vi "Coincidence Stats Rolling Add.vi"(8 "error in (no error)":errorcluster, 10 "New data":T3(array[cluster]), 11 "Rolling array in":T1={"Numofpoints"=10000, "Current index"=0, "Max index"=0, "Data"=[{"initialized array"=[[0, 0, 0, 0, 0, 0, 0, 0, 0, 0, 0, 0], [0, 0, 0, 0, 0, 0, 0, 0, 0, 0, 0, 0], [0, 0, 0, 0, 0, 0, 0, 0, 0, 0, 0, 0], [0, 0, 0, 0, 0, 0, 0, 0, 0, 0, 0, 0], [0, 0, 0, 0, 0, 0, 0, 0, 0, 0, 0, 0], [0, 0, 0, 0, 0, 0, 0, 0, 0, 0, 0, 0], [0, 0, 0, 0, 0, 0, 0, 0, 0, 0, 0, 0], [0, 0, 0, 0, 0, 0, 0, 0, 0, 0, 0, 0], [0, 0, 0, 0, 0, 0, 0, 0, 0, 0, 0, 0], [0, 0, 0, 0, 0, 0, 0, 0, 0, 0, 0, 0], [0, 0, 0, 0, 0, 0, 0, 0, 0, 0, 0, 0], [0, 0, 0, 0, 0, 0, 0, 0, 0, 0, 0, 0]], "Timestamp"=timestamp(0 s since 1904-01-01)}], "Filled"=FALSE}) -> (0 "error out":errorcluster, 2 "Numofpoints":i32, 3 "Rolling array out":T1={"Numofpoints"=10000, "Current index"=0, "Max index"=0, "Data"=[{"initialized array"=[[0, 0, 0, 0, 0, 0, 0, 0, 0, 0, 0, 0], [0, 0, 0, 0, 0, 0, 0, 0, 0, 0, 0, 0], [0, 0, 0, 0, 0, 0, 0, 0, 0, 0, 0, 0], [0, 0, 0, 0, 0, 0, 0, 0, 0, 0, 0, 0], [0, 0, 0, 0, 0, 0, 0, 0, 0, 0, 0, 0], [0, 0, 0, 0, 0, 0, 0, 0, 0, 0, 0, 0], [0, 0, 0, 0, 0, 0, 0, 0, 0, 0, 0, 0], [0, 0, 0, 0, 0, 0, 0, 0, 0, 0, 0, 0], [0, 0, 0, 0, 0, 0, 0, 0, 0, 0, 0, 0], [0, 0, 0, 0, 0, 0, 0, 0, 0, 0, 0, 0], [0, 0, 0, 0, 0, 0, 0, 0, 0, 0, 0, 0], [0, 0, 0, 0, 0, 0, 0, 0, 0, 0, 0, 0]], "Timestamp"=timestamp(0 s since 1904-01-01)}], "Filled"=FALSE}, 5 "Removed elements":T2(array[cluster]))   [LabVIEW 2016]
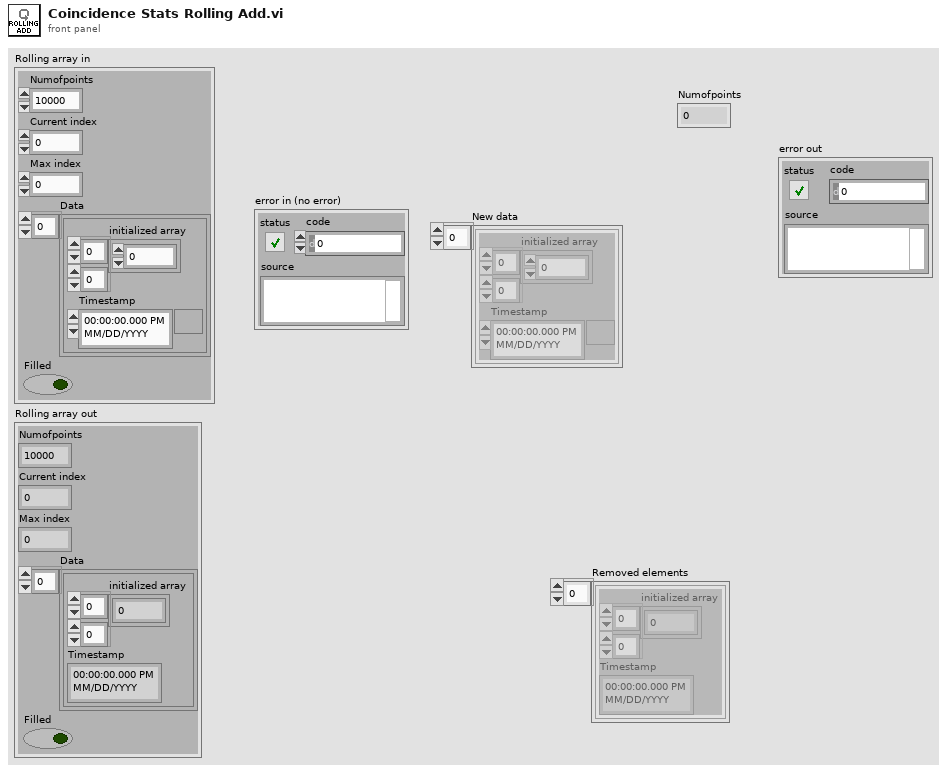
[diagram p1: front panel]
types:
  T1 = cluster{"Numofpoints":i32, "Current index":i32, "Max index":i32, "Data":cluster{"initialized array":i32[][], "Timestamp":timestamp}[], "Filled":bool}
  T2 = cluster{"initialized array":i16[][], "Timestamp":timestamp}[]
  T3 = cluster{"initialized array":i32[][], "Timestamp":timestamp}[]
  T4 = cluster{"initialized array":i32[][], "Timestamp":timestamp}
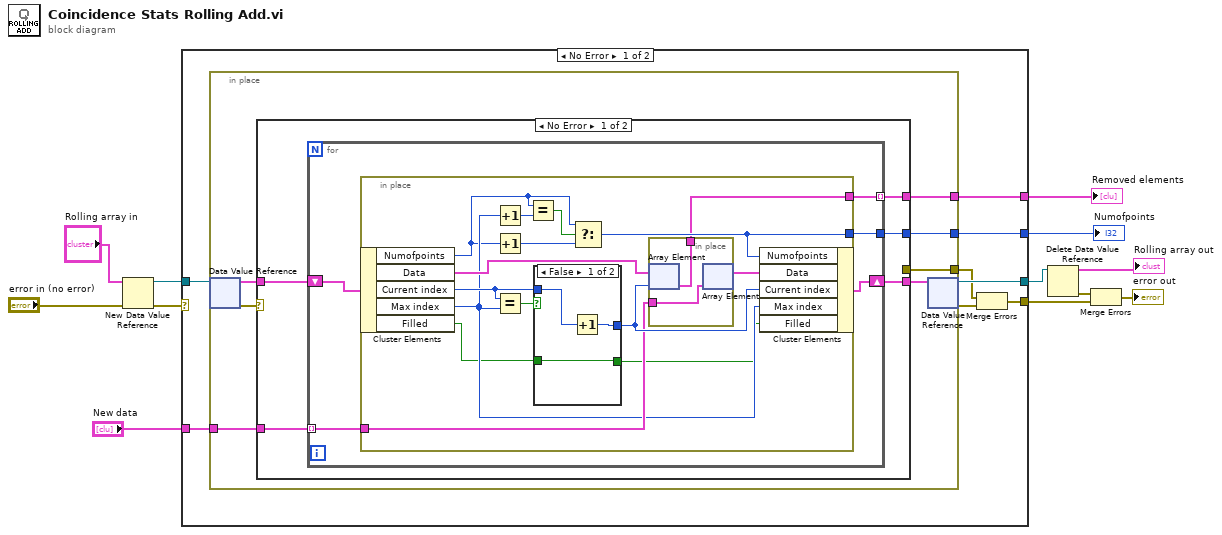
[diagram p0: block diagram]
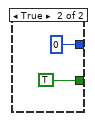
[diagram p2: hidden frame]
diagram:
  n1 = New Data Value Reference(data value="Rolling array in", error in="error in (no error)") -> (data value reference=w12:refnum<data-value>, error out=w9:errorcluster)
  n2 = case shown="No Error" w9 {
    selector: w9 -> [_ w62]
    tunnel: w12 -> [w20 w63]
    tunnel: "New data" -> [w19 _]
    tunnel: [w18 w63] -> w11
    tunnel: [w15 w62] -> w8
    tunnel: [w14 _] -> w5
    tunnel: [w13 _] -> w3
    frame No Error {
      n3 = in-place {
        in-place-border: [w24] -> w17
        in-place-border: w19 -> [w23]
        in-place-border: [w22] -> w14
        in-place-border: [w21] -> w13
        n4 = in-place-dvr #1(w20) -> (w27:T1, w25:errorcluster)
        n5 = case shown="No Error" w25 {
          selector: w25 -> [_ w61]
          tunnel: w27 -> [w32 w60]
          tunnel: [w31 w60] -> w26
          tunnel: [_ w61] -> w24
          tunnel: w23 -> [w30 _]
          tunnel: [w29 _] -> w22
          tunnel: [w28 _] -> w21
          frame No Error {
            n6 = for {
              tunnel: w30 -> [w36] mode=indexing
              shift-right: [w37] -> w31
              shift-left: w32 -> [w34]
              tunnel: [w35] -> w29
              tunnel: [w33] -> w28 mode=indexing
              n7 = in-place {
                in-place-border: w36 -> [w47]
                in-place-border: [w41] -> w35
                in-place-border: [w40] -> w33
                n8 = in-place-cluster #2(w34) -> ("Numofpoints"=w42:i32, "Data"=w52:T3, "Current index"=w51:i32, "Max index"=w46:i32, "Filled"=w39:bool)
                n9 = Increment(x=w46) -> (x+1=w45:i32)
                n10 = Increment(x=w42) -> (x+1=w43:i32)
                n11 = Equal?(x=w51, y=w46) -> (x = y?=w49:bool)
                n12 = Equal?(x=w42, y=w45) -> (x = y?=w44:bool)
                n13 = case shown="False" w49 {
                  tunnel: [w55 0] -> w50
                  tunnel: w51 -> [w54 _]
                  tunnel: w39 -> [w53 _]
                  tunnel: [w53 TRUE] -> w38
                  frame False {
                    n14 = Increment(x=w54) -> (x+1=w55:i32)
                  }
                  frame True {
                  }
                }
                n15 = Select(t=w42, s=w44, f=w43) -> (s? t:f=w41:i32)
                n16 = in-place {
                  in-place-border: w47 -> [w59]
                  in-place-border: [w58] -> w40
                  n17 = in-place-array #3(w52, w50) -> (w58:T4)
                  n18 = in-place-array #3(w59) -> (w48:T3)  [unwired: 1 out]
                }
                n19 = in-place-cluster #2("Numofpoints"=w41, "Data"=w48, "Current index"=w50, "Max index"=w46, "Filled"=w38) -> (w37:T1)
              }
            }
          }
          frame Error {
          }
        }
        n20 = in-place-dvr #1(w26) -> (w18:refnum<data-value>, w16:errorcluster)
      }
      n21 = Merge Errors(w17, w16) -> (w15:errorcluster)
    }
    frame Error {
    }
  }
  "Numofpoints" <- w5
  "Removed elements" <- w3
  n22 = Delete Data Value Reference(data value reference=w11) -> (data value=→"Rolling array out":T1, error out=w7:errorcluster)  [unwired: 1 in]
  n23 = Merge Errors(w7, w8) -> (→"error out":errorcluster)
